vi "simple 1.vi"() -> ()   [LabVIEW 2022 SP3]
panel:
  out "Result":dbl
  in  "Number 2":dbl
  in  "Number 1":dbl
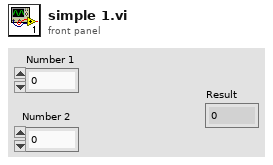
[diagram p1: front panel]
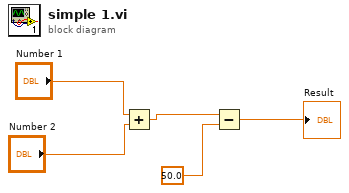
[diagram p0: block diagram]
diagram:
  n1 = Add(x="Number 1", y="Number 2") -> (x+y=w5:dbl)
  n2 = Subtract(x=w5, y=50.0) -> (x-y=→"Result":dbl)
